vi "Predict.vi"(8 "error in (no error)":errorcluster, 9 "Length":i32=4, 10 "Candidate Map":map{i32, string[][]}(c390), 11 "MarkovModel in":refnum<class "MarkovModel.lvclass">) -> (0 "error out":errorcluster, 2 "Winners":cluster{"Class Name":string, "Count":i32}[](array[cluster]), 3 "MarkovModel out":refnum<class "MarkovModel.lvclass">)   [LabVIEW 2020, in "MarkovModel.lvclass"]
uses:
  MarkovModel.lvclass
  MarkovModel.lvclass/MarkovModel.ctl
  <vilib>/Utility/miscctls.llb/LVMapReplaceAction.ctl
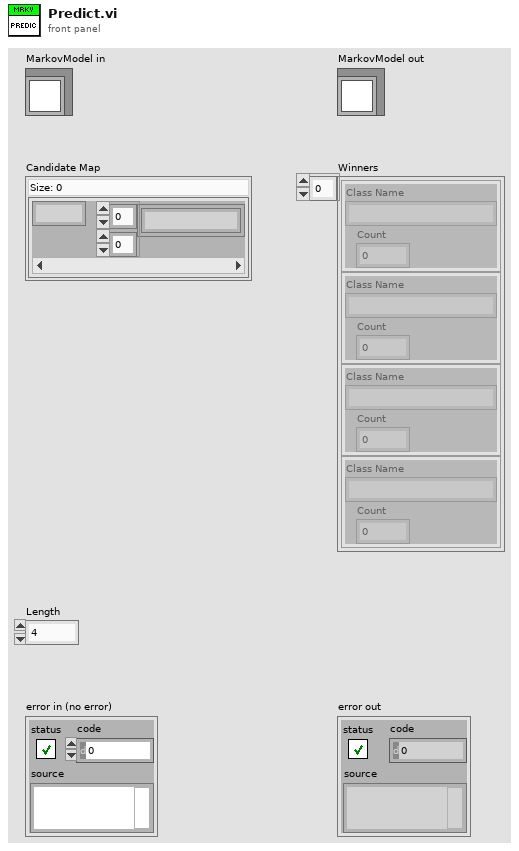
[diagram p1: front panel]
types:
  T1 = map{string[], cluster{"Class Name":string, "Count":i32}[]}
  T2 = typedef "LVMapReplaceAction.ctl" = enum32{"Modify Entry only if found", "Add or Modify Entry", "Delete Entry"}
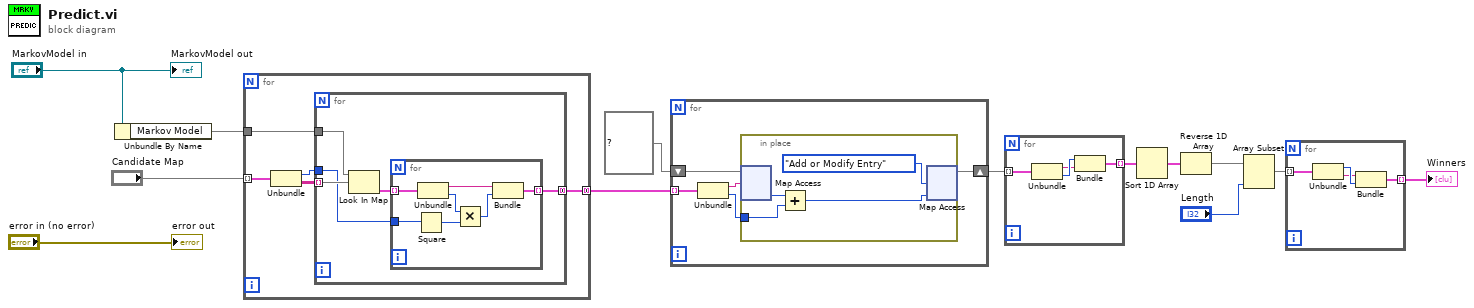
[diagram p0: block diagram]
diagram:
  n1 = Unbundle By Name("MarkovModel in") -> ("Markov Model"=w10:T1)
  n2 = for {
    tunnel: w10 -> [w18]
    tunnel: [w17] -> w2 mode=concatenating
    tunnel: "Candidate Map" -> [w16] mode=indexing
    n3 = Unbundle(w16) -> ("Order"=w14:i32, "Candidates"=w15:string[][])
    n4 = for {
      tunnel: w18 -> [w22]
      tunnel: [w19] -> w17 mode=concatenating
      tunnel: w15 -> [w23] mode=indexing
      tunnel: w14 -> [w20]
      n5 = Look In Map(map=w22, key=w23) -> (value=w21:cluster{"Class Name":string, "Count":i32}[])  [unwired: 1 in, 1 out]
      n6 = for {
        tunnel: w21 -> [w30] mode=indexing
        tunnel: w20 -> [w28]
        tunnel: [w24] -> w19 mode=indexing
        n7 = Square(x=w28) -> (x^2=w26:i32)
        n8 = Unbundle(w30) -> ("Class Name"=w29:string, "Count"=w27:i32)
        n9 = Multiply(x=w27, y=w26) -> (x*y=w25:i32)
        n10 = Bundle("Class Name"=w29, w25) -> (w24:cluster{"Class Name":string, i32})  [unwired: 1 in]
      }
    }
  }
  n11 = for {
    tunnel: w2 -> [w35] mode=indexing
    shift-right: [w31] -> w4
    shift-left: map{string, i32} {} ("Map") -> [w32]
    n12 = Unbundle(w35) -> ("Class Name"=w34:string, w33:i32)
    n13 = in-place {
      in-place-border: w33 -> [w37]
      n14 = in-place-map #1(w32, w34) -> (w38:i32)  [unwired: 1 in, 1 out]
      n15 = Add(x=w38, y=w37) -> (x+y=w36:i32)
      n16 = in-place-map #1(w36, LVMapReplaceAction."Add or Modify Entry" ("action")) -> (w31:map{string, i32})  [unwired: 2 out]
    }
  }
  n17 = for {
    tunnel: w4 -> [w43] mode=indexing
    tunnel: [w40] -> w5 mode=indexing
    n18 = Unbundle(w43) -> (w41:string, w42:i32)
    n19 = Bundle(w42, w41) -> (w40:cluster{i32, string})  [unwired: 1 in]
  }
  n20 = Sort 1D Array(array=w5) -> (sorted array=w7:cluster{i32, string}[])
  n21 = Reverse 1D Array(array=w7) -> (reversed array=w8:cluster{i32, string}[])
  n22 = Array Subset(array=w8, length="Length") -> (w6:cluster{i32, string}[])  [unwired: 1 in]
  n23 = for {
    tunnel: w6 -> [w47] mode=indexing
    tunnel: [w44] -> w9 mode=indexing
    n24 = Unbundle(w47) -> (w46:i32, w45:string)
    n25 = Bundle(w45, w46) -> (w44:cluster{string, i32})  [unwired: 1 in]
  }
  "Winners" <- w9
  "error out" <- "error in (no error)"
  "MarkovModel out" <- "MarkovModel in"
